vi "Read Customer.vi"(8 "error in (no error)":errorcluster, 11 "Order in":refnum<class "Order.lvclass">) -> (0 "error out":errorcluster, 2 "Customer":refnum<class "Customer.lvclass">, 3 "Order out":refnum<class "Order.lvclass">)   [LabVIEW 2020, in "Order.lvclass"]
doc: "Simple accessor method to read the Customer enqueuer."
uses:
  Order.lvclass
  Processes/People/Customers/Customer/Customer.lvclass
  Order.lvclass/Order.ctl
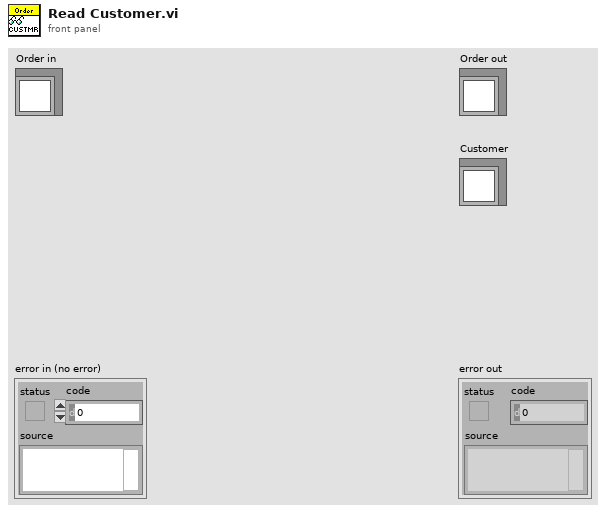
[diagram p1: front panel]
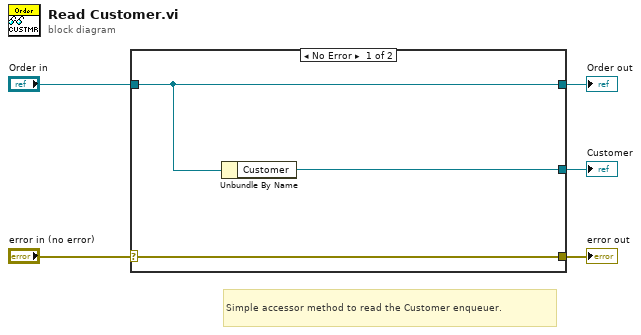
[diagram p0: block diagram]
diagram:
  # "Simple accessor method to read the Customer enqueuer."
  n1 = case shown="No Error" "error in (no error)" {
    selector: "error in (no error)" -> [w8 w9]
    tunnel: [w8 w9] -> w4
    tunnel: [w7 w10] -> w2
    tunnel: "Order in" -> [w7 w10]
    tunnel: [w6 _] -> w1
    frame No Error {
      n2 = Unbundle By Name(w7) -> ("Customer"=w6:refnum<class "Customer.lvclass">)
    }
    frame Error {
    }
  }
  "error out" <- w4
  "Order out" <- w2
  "Customer" <- w1
